vi "Test Method Status Reset on Start.vi"(8 "error in (no error)":errorcluster, 11 "Result Model Result Recording Test in":refnum<class "Result Model Result Recording Test.lvclass">) -> (0 "error out":errorcluster, 3 "Result Model Result Recording Test out":refnum<class "Result Model Result Recording Test.lvclass">)   [LabVIEW 2020, in "Result Model Result Recording Test.lvclass"]
uses:
  Result Model Result Recording Test.lvclass
  C:/Program Files (x86)/National Instruments/LabVIEW 2020/vi.lib/Astemes/LUnit/Test Case.lvclass
  source/Core/Result/Result.ctl
  source/Core/Result/Status.ctl
  source/Core/Result/Type.ctl
  <vilib>/Astemes/LUnit/Test Case.lvclass/Test Case.ctl
  ae2c71b8-32bb-49d1-8500-0119bfec74ff.vi
  <vilib>/Astemes/LUnit/Append Pass Result.vi
  <vilib>/Astemes/LUnit/Append Fail Result.vi
  <vilib>/Astemes/LUnit/Describe Comparison.vi
  <vilib>/Astemes/LUnit/Compare Variants.vi
  <vilib>/Astemes/LUnit/Variant to string.vi
  <vilib>/Utility/Data Type/Get Type Information.vi
  <vilib>/Utility/LVClass/Get LV Class Name.vi
  source/User Interface/Result Model by Reference/Result Model by Reference.lvclass
  Result Model Result Recording Test.lvclass/Result Model Result Recording Test.ctl
  source/Core/Result/Result.lvlib
  source/User Interface/Result Model/Tree Item Filter.ctl
  source/User Interface/Result Model/Result Model.lvclass
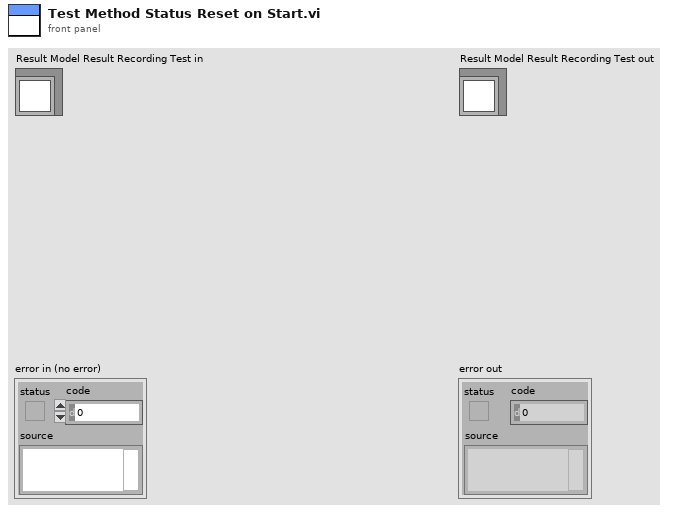
[diagram p1: front panel]
types:
  T1 = typedef "Result Model.lvclass/Tree Item Filter.ctl" = enum16{"All", "Only Fails"}
  T2 = typedef "Result.lvlib/Result.ctl" = cluster{"Name":string, "Message":string, "Description":string, "Status":T3, "Result Type":T4, "Execution Time":dbl}
  T3 = typedef "Result.lvlib/Status.ctl" = enum16{"", "Passed", "Failed", "Error", "Skipped", "Setup Error", "Broken", "Teardown Error"}
  T4 = typedef "Result.lvlib/Type.ctl" = enum16{"Test Case", "Test Suite", "Test Run", "Pass", "Fail", "Skip", "Pass if", "Fail if", "Pass if Error", "Fail if Error", "Pass if Equal", "Fail if Equal"}
  T5 = cluster{"Left Cell String":string, "Child Text":string[], "Child Tag":string, "Item Indent":i32, "Child Only?":bool, "Glyph Index":i32}[]
  T6 = cluster{"Left Cell String":string, "Child Text":string[], "Child Tag":string, "Item Indent":i32, "Child Only?":bool, "Glyph Index":i32}
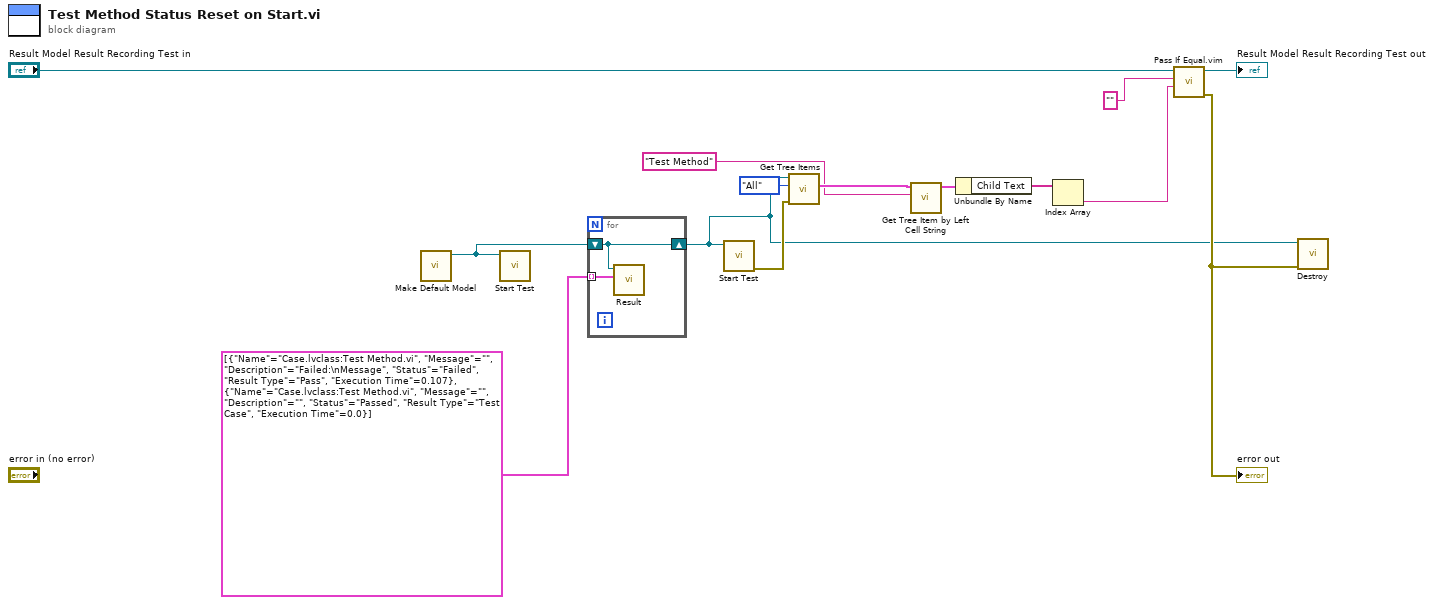
[diagram p0: block diagram]
diagram:
  n1 = call "Make Default Model.vi"() -> ("Result Model out"=w3:refnum<class "Result Model by Reference.lvclass">)  [unwired: 10 in, 1 out]
  n2 = call "Start Test.vi"("Result Model In"=w3) -> ()  [unwired: 10 in, 1 out]
  n3 = for {
    tunnel: T2[] [{"Name"="Case.lvclass:Test Method.vi", "Message"="", "Description"="Failed:\nMessage", "Status"=enum."Failed", "Result Type"=enum."Pass", "Execution Time"=0.107}, {"Name"="Case.lvclass:Test Method.vi", "Message"="", "Description"="", "Status"=enum."Passed", "Result Type"=enum."Test Case", "Execution Time"=0.0}] ("Results") -> [w16] mode=indexing
    shift-right: [w15] -> w1
    shift-left: w3 -> [w15]
    n4 = call-dynamic "Result.vi"("Results"=w16, "Result Model by Reference In"=w15) -> ()  [unwired: 9 in, 1 out]
  }
  n5 = call "Start Test.vi"("Result Model In"=w1) -> ("error out"=w2:errorcluster)  [unwired: 10 in]
  n6 = call "Get Tree Items.vi"("error in (no error)"=w2, "Filter"=Tree_Item_Filter."All", "Result Model by Reference In"=w1) -> ("Tree Items"=w11:T5)  [unwired: 7 in, 1 out]
  n7 = call "Get Tree Item by Left Cell String.vi"("Left Cell String"="Test Method" ("Item"), "Tree Items"=w11) -> ("Item"=w9:T6)  [unwired: 9 in]
  n8 = Unbundle By Name(w9) -> ("Child Text"=w8:string[])
  n9 = Index Array(array=w8) -> (element=w7:string)  [unwired: 1 in]
  n10 = call "Pass If Equal.vim"("Actual"=w7, "Expected"="" ("element"), "LUnit Test Case In"="Result Model Result Recording Test in") -> ("error out"=w4:errorcluster, "LUnit Test Case Out"=→"Result Model Result Recording Test out":refnum<class "Result Model Result Recording Test.lvclass">)  [unwired: 7 in]
  "error out" <- w4
  n11 = call "Destroy.vi"("error in (no error)"=w4, "Result Model in"=w1) -> ()  [unwired: 9 in, 1 out]
